vi "ProdaNG.File.Export.TP.vi"(5 "Identification":T3, 6 "reason":string, 7 "TestStepsTree":refnum<vi>, 8 "error in (no error)":errorcluster, 9 "Idx":i32, 10 "TS":T1, 11 "dbHandleIn":i32) -> (0 "error out":errorcluster, 3 "dbHandle":i32)   [LabVIEW 2016]
uses:
  ProdaNG.File.Step.ctl
  ProdaNG.Tree.Fglb.Value.ctl
  ProdaNG.Tree.Fglb.Action.ctl
  ProdaNG.Tree.Fglb.Data.ctl
  ProdaNG.Tree.Fglb.Element.ctl
  ProdaNG.Configurator.Glb.vi
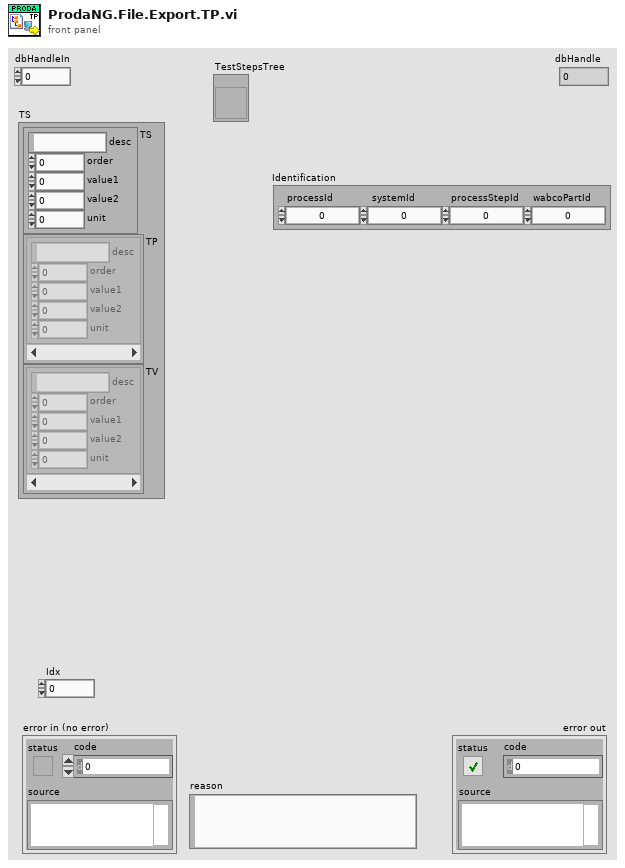
[diagram p1: front panel]
types:
  T1 = typedef "ProdaNG.File.Step.ctl" = cluster{"TS":T2, "TP":T2[], "TV":T2[]}
  T2 = typedef "ProdaNG.Tree.Fglb.Value.ctl" = cluster{"desc":string, "order":i32, "value1":dbl, "value2":dbl, "unit":i32}
  T3 = cluster{"processId":i32, "systemId":i32, "processStepId":i32, "wabcoPartId":i32}
  T4 = typedef "ProdaNG.Tree.Fglb.Data.ctl" = cluster{"tag":string, "row":i32, "element":T5, "idx1":i32, "idx2":i32, "file":bool}
  T5 = typedef "ProdaNG.Tree.Fglb.Element.ctl" = enum16{"-", "PP", "TS", "TP", "TV"}
  T6 = typedef "ProdaNG.Tree.Fglb.Action.ctl" = enum16{"init", "add", "get by row", "get by tag", "get by idx"}
  T7 = typedef "ProdaNG.TestStep.ctl" = cluster{"i_id":i32, "processStepId":i32, "testSequence":i32, "testOrder":i32, "mdReason":string, "mdUser":string, "mdTime":string, "description":string}
  T8 = typedef "ProdaNG.TestStepParam.ctl" = cluster{"i_id":i32, "testStepId":i32, "unitId":i32, "contentId":string, "previewId":string, "value":dbl, "valueText":string, "paramSequence":i32, "history":i32, "mdReason":string, "mdUser":string, "mdTime":string, "description":string}
  T9 = typedef "ProdaNG.TestValue.ctl" = cluster{"i_id":i32, "testStepId":i32, "releaseId":i32, "unitId":i32, "contentId":string, "previewId":string, "maximum":dbl, "minimum":dbl, "valueText":string, "testValueSequence":i32, "history":i32, "mdReason":string, "mdUser":string, "mdTime":string, "description":string}
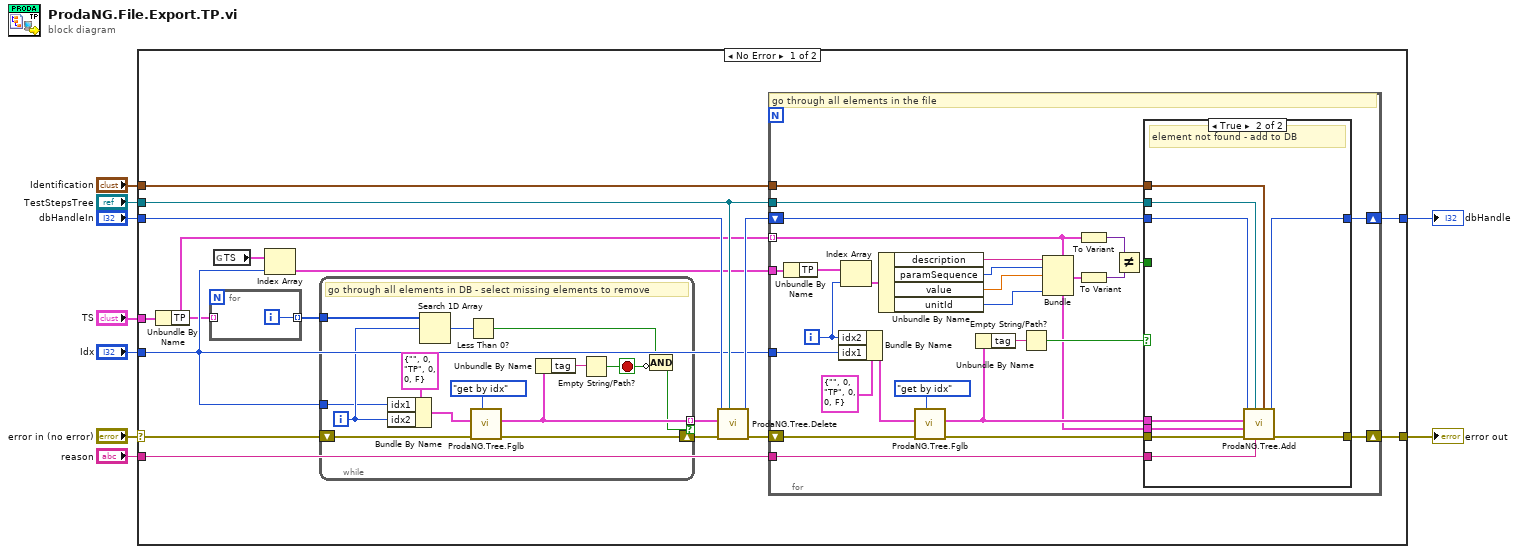
[diagram p0: block diagram]
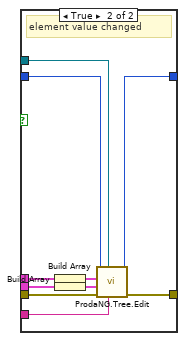
[diagram p3: hidden frame]
diagram:
  n1 = case shown="No Error" "error in (no error)" {
    selector: "error in (no error)" -> [w24 w101]
    tunnel: [w16 w101] -> w9
    tunnel: "dbHandleIn" -> [w19 w100]
    tunnel: [w26 w100] -> w6
    tunnel: "TS" -> [w25 _]
    tunnel: "reason" -> [w17 _]
    tunnel: "Identification" -> [w15 _]
    tunnel: "TestStepsTree" -> [w14 _]
    tunnel: "Idx" -> [w11 _]
    frame No Error {
      n2 = Unbundle By Name(w25) -> ("TP"=w10:T2[])
      n3 = for {
        tunnel: w10 -> [_] mode=indexing
        tunnel: [w27] -> w23 mode=indexing
        i -> [w27]
      }
      n4 = global read "ProdaNG.Configurator.Glb.vi" "TS"() -> (w13:cluster{"TS":T7, "TP":T8[], "TV":T9[]}[])
      n5 = Index Array(array=w13, index=w11) -> (element=w12:cluster{"TS":T7, "TP":T8[], "TV":T9[]})
      n6 = while {
        tunnel: [w37] -> w20 mode=indexing if=w33
        shift-right: [w36] -> w22
        shift-left: w24 -> [w40]
        tunnel: w23 -> [w35]
        tunnel: w11 -> [w29]
        i -> [w30]
        stop <- w28 stop-if-true
        # "go through all elements in DB - select missing elements to remove"
        n7 = Bundle By Name(cluster=T4 {"tag"="", "row"=0, "element"=enum."TP", "idx1"=0, "idx2"=0, "file"=FALSE} ("entry in"), "idx1"=w29, "idx2"=w30) -> (w31:T4)
        n8 = Search 1D Array(1D array=w35, element=w30) -> (index of element=w34:i32)  [unwired: 1 in]
        n9 = Less Than 0?(x=w34) -> (x < 0?=w32:bool)
        n10 = call "ProdaNG.Tree.Fglb.vi"("Action (add)"=ProdaNG.Tree.Fglb.Action."get by idx", "error in"=w40, "entry in"=w31) -> ("error out"=w36:errorcluster, "found entry"=w37:T4)  [unwired: 6 in, 1 out]
        n11 = Unbundle By Name(w37) -> ("tag"=w38:string)
        n12 = Empty String/Path?(string/path=w38) -> (empty?=w28:bool)
        n13 = Compound Arithmetic op=AND(w32, invert w28) -> (w33:bool)
      }
      n14 = call "ProdaNG.Tree.Delete.vi"("TestStepsTree"=w14, "error in (no error)"=w22, "Elements to delete"=w20, "dbHandleIn"=w19) -> ("error out"=w21:errorcluster, "dbHandle"=w18:i32)  [unwired: 6 in]
      n15 = for {
        shift-right: [w61] -> w16
        shift-left: w21 -> [w66]
        shift-right: [w58] -> w26
        shift-left: w18 -> [w62]
        tunnel: w10 -> [w42] mode=indexing
        tunnel: w17 -> [w59]
        tunnel: w15 -> [w56]
        tunnel: w14 -> [w55]
        tunnel: w12 -> [w46]
        tunnel: w11 -> [w44]
        i -> [w43]
        # "go through all elements in the file"
        n16 = Unbundle By Name(w46) -> ("TP"=w45:T8[])
        n17 = Bundle By Name(cluster=T4 {"tag"="", "row"=0, "element"=enum."TP", "idx1"=0, "idx2"=0, "file"=FALSE} ("entry in"), "idx2"=w43, "idx1"=w44) -> (w67:T4)
        n18 = Index Array(array=w45, index=w43) -> (element=w57:T8)
        n19 = Unbundle By Name(w57) -> ("description"=w54:string, "paramSequence"=w53:i32, "value"=w52:dbl, "unitId"=w51:i32)
        n20 = call "ProdaNG.Tree.Fglb.vi"("Action (add)"=ProdaNG.Tree.Fglb.Action."get by idx", "error in"=w66, "entry in"=w67) -> ("error out"=w63:errorcluster, "found entry"=w60:T4)  [unwired: 6 in, 1 out]
        n21 = Unbundle By Name(w60) -> ("tag"=w65:string)
        n22 = Empty String/Path?(string/path=w65) -> (empty?=w64:bool)
        n23 = Bundle(cluster=w42, "desc"=w54, "order"=w53, "value1"=w52, "unit"=w51) -> (w50:T2)  [unwired: 1 in]
        n24 = To Variant(anything=w42) -> (Variant=w49:variant)
        n25 = To Variant(anything=w50) -> (Variant=w48:variant)
        n26 = Not Equal?(x=w49, y=w48) -> (x != y?=w47:bool)
        n27 = case shown="True" w64 {
          tunnel: w63 -> [w78 w99]
          tunnel: w62 -> [w74 w98]
          tunnel: [w77 w93] -> w61
          tunnel: w60 -> [w75 w97]
          tunnel: w42 -> [w72 w96]
          tunnel: w59 -> [w76 w95]
          tunnel: [w73 w94] -> w58
          tunnel: w56 -> [_ w92]
          tunnel: w55 -> [w71 w91]
          tunnel: w47 -> [w70 _]
          frame False {
            # "element found"
            n28 = case shown="False" w70 {
              tunnel: w78 -> [w80 w90]
              tunnel: [w80 w89] -> w77
              tunnel: w76 -> [_ w88]
              tunnel: w75 -> [_ w87]
              tunnel: w74 -> [w79 w85]
              tunnel: [w79 w84] -> w73
              tunnel: w72 -> [_ w83]
              tunnel: w71 -> [_ w81]
              frame False {
              }
              frame True {
                # "element value changed"
                n29 = Build Array(w87) -> (w86:T4[])
                n30 = Build Array(w83) -> (w82:T2[])
                n31 = call "ProdaNG.Tree.Edit.vi"("reason"=w88, "TestStepsTree"=w81, "error in (no error)"=w90, "Selected elements values"=w82, "Selected elements"=w86, "dbHandleIn"=w85) -> ("error out"=w89:errorcluster, "dbHandle"=w84:i32)  [unwired: 4 in]
              }
            }
          }
          frame True {
            # "element not found - add to DB"
            n32 = call "ProdaNG.Tree.Add.vi"("Identification"=w92, "reason"=w95, "TestStepsTree"=w91, "error in (no error)"=w99, "Element values"=w96, "Element to add"=w97, "dbHandleIn"=w98) -> ("error out"=w93:errorcluster, "dbHandle"=w94:i32)  [unwired: 3 in]
          }
        }
      }
    }
    frame Error {
    }
  }
  "error out" <- w9
  "dbHandle" <- w6
